vi "PCSMain.get i attribute.vi"(0 "i ref in":refnum<vi>, 5 "error in (no error)":errorcluster) -> (14 "i ref out":refnum<vi>, 16 "i attribute":T1, 19 "error out":errorcluster)   [LabVIEW 2014, in "PCSMain.lvlib"]
doc: "Gets the i attribute data of an object.\n\nLicense Agreement for this software:\n\nCopyright (C)\nGesellschaft für Schwerionenforschung, GSI\nPlanckstr. 1\n64291 Darmstadt\nGermany\n\nContact: D.Beck@gsi.de \n\nThis program is free software; you can redistribute it and/or modify it under the terms of the GNU General Public License as published by the Free Software Foundation; either version 2 of the license, or (at your option) any later version.\n\nThis program is distributed in the hope that it will be useful, but WITHOUT ANY WARRANTY; without even the implied warranty of MERCHANTABILITY or FITNESS FOR A PARTICULAR PURPOSE. See the GNU General License for more details (http://www.gnu.org).\n\nGesellschaft für Schwerionenforschung, GSI\nPlanckstr. 1, 64291 Darmstadt, Germany\nFor all questions and ideas contact: M.Richter@gsi.de, H.Brand@gsi.de or D.Beck@gsi.de.\nLast update: 17-JUN-2004"
uses:
  PCSMain.lvlib
  PCSMain.i attribute.ctl
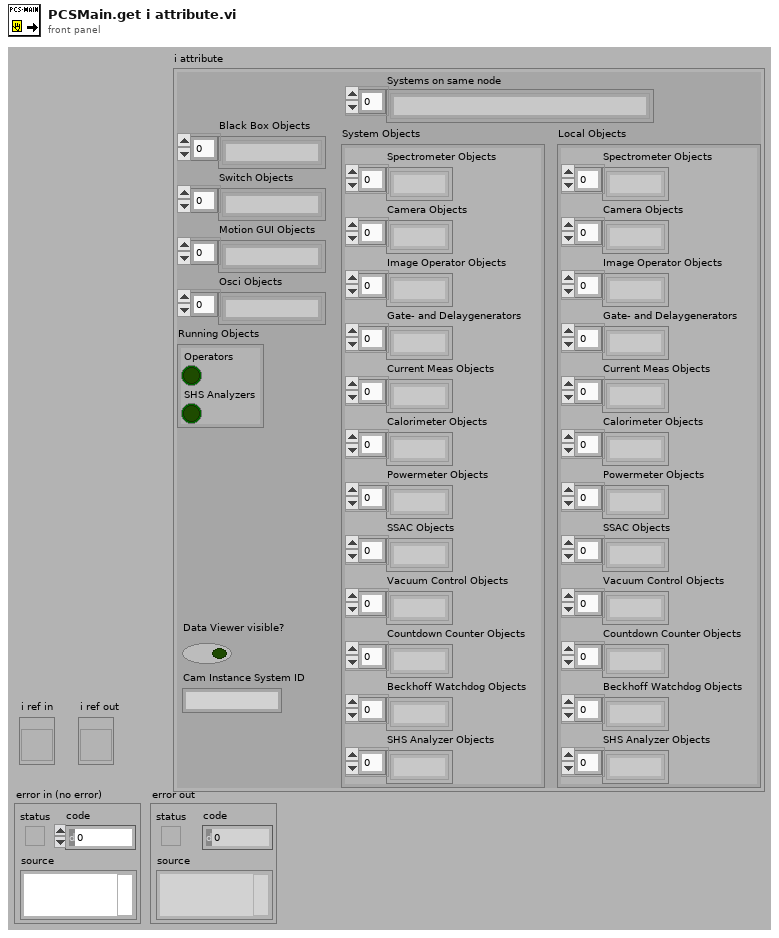
[diagram p1: front panel]
types:
  T1 = typedef "PCSMain.lvlib/PCSMain.i attribute.ctl" = cluster{"System Objects":cluster{"Spectrometer Objects":string[], "Camera Objects":string[], "Image Operator Objects":string[], "Gate- and Delaygenerators":string[], "Current Meas Objects":string[], "Calorimeter Objects":string[], "Powermeter Objects":string[], "SSAC Objects":string[], "Vacuum Control Objects":string[], "Countdown Counter Objects":string[], "Beckhoff Watchdog Objects":string[], "SHS Analyzer Objects":string[]}, "Local Objects":cluster{"Spectrometer Objects":string[], "Camera Objects":string[], "Image Operator Objects":string[], "Gate- and Delaygenerators":string[], "Current Meas Objects":string[], "Calorimeter Objects":string[], "Powermeter Objects":string[], "SSAC Objects":string[], "Vacuum Control Objects":string[], "Countdown Counter Objects":string[], "Beckhoff Watchdog Objects":string[], "SHS Analyzer Objects":string[]}, "Systems on same node":string[], "Data Viewer visible?":bool, "Running Objects":cluster{"Operators":bool, "SHS Analyzers":bool}, "Cam Instance System ID":string, "Black Box Objects":string[], "Switch Objects":string[], "Motion GUI Objects":string[], "Osci Objects":string[]}
  T2 = enum16{"SetAttribute", "GetAttribute", "CreateAttribute", "DestroyAttribute", "DestroyAllAtributes"}
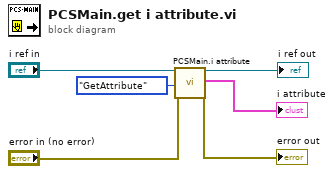
[diagram p0: block diagram]
diagram:
  n1 = call "PCSMain.i attribute.vi"("VI Refnum"="i ref in", "Action"=T2."GetAttribute", "error in (no error)"="error in (no error)") -> ("VI Refnum out"=→"i ref out":refnum<vi>, "CLASS.i attribute out"=→"i attribute":T1, "error out"=→"error out":errorcluster)  [unwired: 14 in]
